vi "位置属性控制.vi"() -> ()   [LabVIEW 2010]
panel:
  in  "赛马速度":u8(slide) scale=0.0..200.0
  in  "停止":bool
  out "图片下拉列表":u16(ring)
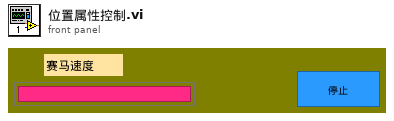
[diagram p1: front panel]
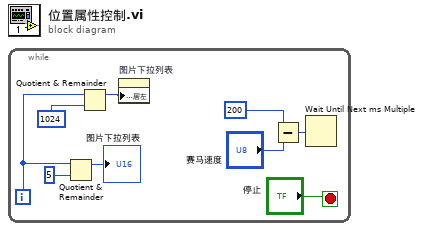
[diagram p0: block diagram]
diagram:
  n1 = while {
    i -> [w7]
    stop <- "停止" stop-if-true
    n2 = Quotient & Remainder(x=w7, y=5) -> (x-y*floor(x/y)=→"图片下拉列表":i32)  [unwired: 1 out]
    n3 = Quotient & Remainder(x=w7, y=1024) -> (x-y*floor(x/y)=w5:i32)  [unwired: 1 out]
    n4 = property on="图片下拉列表" class="Ring (严格)"("位置:居左"=w5) -> ()  [unwired: 2 in, 2 out]
    n5 = Subtract(x=200, y="赛马速度") -> (x-y=w2:i32)
    n6 = Wait Until Next ms Multiple(millisecond multiple=w2) -> ()  [unwired: 1 out]
  }
